vi "PmodGYRORead.vi"(7 "I2C Channel (0)":u8, 8 "error in (no error)":errorcluster, 9 "Resolution (dps)":enum16{"2000", "500", "250"}(ring), 10 "Address":enum8{"0x68", "0x69"}(ring)=enum."0x69", 11 "LINX Resource in":T1) -> (0 "error out":errorcluster, 2 "Gyro XYZ (degrees/sec)":cluster{"X":i16, "Y":i16, "Z":i16}, 3 "LINX Resource out":T1)   [LabVIEW 2018]
doc: "Point the I2C to the 0x28 register with a 1 in the MSb slot to configure the device to read more than one byte at a time, thus 0xA8 is used.\n\nRead 6 bytes from register 0x28 and the subsequent registers. Combine the x, y, and z bytes and convert to a 2's complement signed 16 bit integer. Multiply by the corresponding resolution to get the correct gyro reading.\n\nThis VI outputs the Gyro x, y, and z values in degrees per second."
uses:
  <vilib>/MakerHub/LINX/Private/Type Defs/Platform.ctl
  <vilib>/MakerHub/LINX/Private/Type Defs/Interface.ctl
  <vilib>/MakerHub/LINX/Private/Device/Type Defs/TCP Config.ctl
  <vilib>/MakerHub/LINX/Private/Device/Type Defs/Channels.ctl
  <vilib>/MakerHub/LINX/Private/Device/Type Defs/LINX Device Config.ctl
  <vilib>/MakerHub/LINX/Private/Type Defs/LINX Ref.ctl
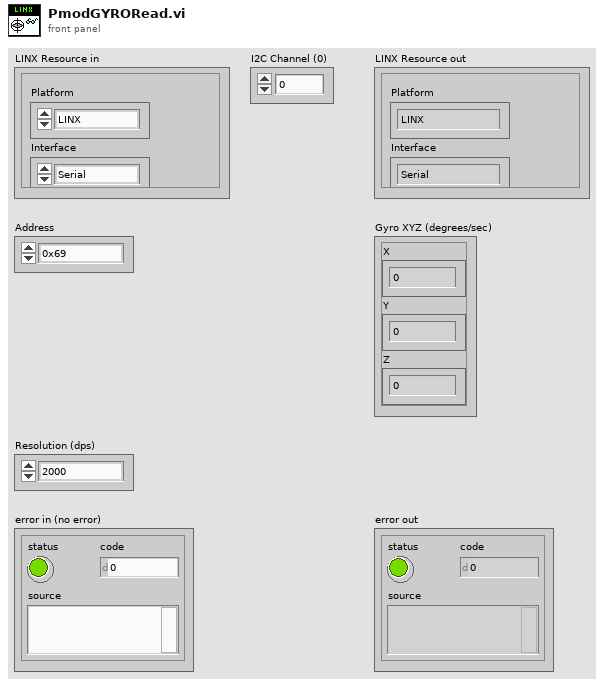
[diagram p1: front panel]
types:
  T1 = typedef "LMH-LINX.lvlib/LINX Ref.ctl" = cluster{"Platform":T2, "Interface":T3, "LINX Device Config":T4}
  T2 = typedef "LMH-LINX.lvlib/Platform.ctl" = enum16{"LINX", "myRIO"}
  T3 = typedef "LMH-LINX.lvlib/Interface.ctl" = enum16{"Serial", "TCP"}
  T4 = typedef "LMH-LINX.lvlib/Device.lvlib/LINX Device Config.ctl" = cluster{"Interface":T3, "COM Port":refnum<visa-resource-name>, "TCP Configuration":T5, "Device Family":u8, "Device ID":u8, "Device Name":string, "TCP Ref":refnum<k5>, "Channels":T6}
  T5 = typedef "LMH-LINX.lvlib/Device.lvlib/TCP Config.ctl" = cluster{"IP Address":string, "Port":u16}
  T6 = typedef "LMH-LINX.lvlib/Channels.ctl" = cluster{"DI":u8[], "DO":u8[], "AI":u8[], "AO":u8[], "PWM":u8[], "QE":u8[], "UART":u8[], "I2C 2":u8[], "SPI":u8[], "CAN":u8[], "Servo":u8[], "AI Ref (V)":dbl, "AO Ref (V)":dbl, "AO Resolution (Bits)":u8}
  T7 = cluster{"Decimal I16":i16, "Decimal I16":i16, "Decimal I16":i16}
  T8 = cluster{"Decimal I16":dbl, "Decimal I16":dbl, "Decimal I16":dbl}
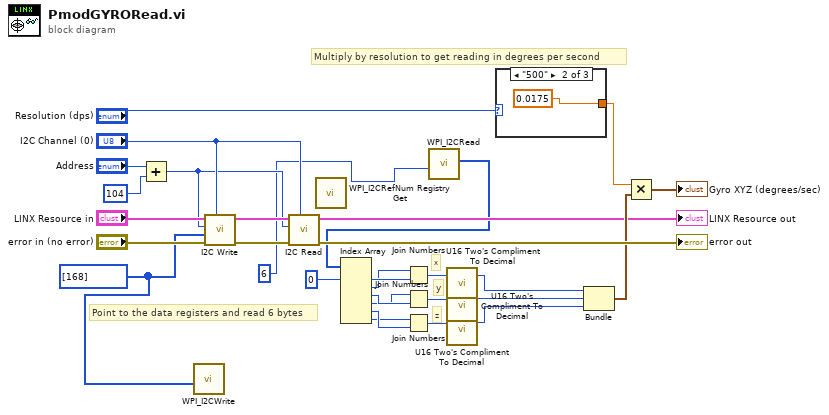
[diagram p0: block diagram]
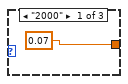
[diagram p2: hidden frame]
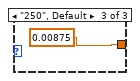
[diagram p3: hidden frame]
diagram:
  w1 = u8[] [168] ("Data")
  # "Multiply by resolution to get reading in degrees per second"
  # "Point to the data registers and read 6 bytes"
  # "z"
  # "y"
  # "x"
  n1 = Add(x="Address", y=u8 104) -> (x+y=w10:u8)
  n2 = call <vilib>:"WPI_I2CWrite.vi"("I2CDataToSend"=w1) -> ()  [unwired: 9 in, 2 out]
  n3 = call <vilib>:"I2C Write.vi"("I2C Channel"="I2C Channel (0)", "Error In"="error in (no error)", "Data"=w1, "I2C Slave Address (0)"=w10, "LINX Resource"="LINX Resource in") -> ("Error Out"=w14:errorcluster, "LINX Resource"=w16:T1)  [unwired: 5 in]
  n4 = call <vilib>:"I2C Read.vi"("I2C Channel"="I2C Channel (0)", "Error In"=w14, "I2C Slave Address (0)"=w10, "LINX Resource"=w16) -> ("Error Out"=→"error out":errorcluster, "LINX Resource"=→"LINX Resource out":T1)  [unwired: 5 in, 1 out]
  n5 = call <vilib>:"WPI_I2CRefNum Registry Get.vi"() -> ()  [unwired: 10 in, 2 out]
  n6 = call <vilib>:"WPI_I2CRead.vi"("I2CBytesToRead"=u8 6 ("Bytes To Read")) -> ("Data Out"=w3:u8[])  [unwired: 8 in, 2 out]
  n7 = Index Array(array=w3, index #1=0 ("index")) -> (element #1=w9:u8, element #2=w8:u8, element #3=w7:u8, element #4=w6:u8, element #5=w5:u8, element #6=w4:u8)  [unwired: 5 in]
  n8 = Join Numbers(hi=w8, lo=w9) -> ((hi.lo)=w20:u16)
  n9 = Join Numbers(hi=w6, lo=w7) -> ((hi.lo)=w22:u16)
  n10 = Join Numbers(hi=w4, lo=w5) -> ((hi.lo)=w21:u16)
  n11 = call <vilib>:"U16 Two's Compliment To Decimal.vi"("Two's Compliment U16"=w20) -> ("Decimal I16"=w23:i16)  [unwired: 2 in]
  n12 = call <vilib>:"U16 Two's Compliment To Decimal.vi"("Two's Compliment U16"=w22) -> ("Decimal I16"=w24:i16)  [unwired: 2 in]
  n13 = call <vilib>:"U16 Two's Compliment To Decimal.vi"("Two's Compliment U16"=w21) -> ("Decimal I16"=w25:i16)  [unwired: 2 in]
  n14 = case shown="\"500\"" "Resolution (dps)" {
    tunnel: [0.07 0.0175 0.00875] -> w27
    frame "2000" {
    }
    frame "500" {
    }
    frame "250", Default {
    }
  }
  n15 = Bundle("Decimal I16"=w23, "Decimal I16"=w24, "Decimal I16"=w25) -> (w26:T7)  [unwired: 1 in]
  n16 = Multiply(x=w27, y=w26) -> (x*y=→"Gyro XYZ (degrees/sec)":T8)
